vi "MBDRV_Operation.vi"(7 "Unit Address (1)":u8=1, 8 "error in (no error)":errorcluster, 10 "Command List":T4, 11 "VISA resource name":refnum<visa-resource-name>) -> (0 "error out":errorcluster, 2 "Response List":T1, 3 "VISA resource name out":refnum<visa-resource-name>)   [LabVIEW 2010]
uses:
  MBDRV_Command List.ctl
  MBDRV_Command Data.ctl
  MBDRV_Action.ctl
  MBDRV_Response List.ctl
  MBDRV_Response.ctl
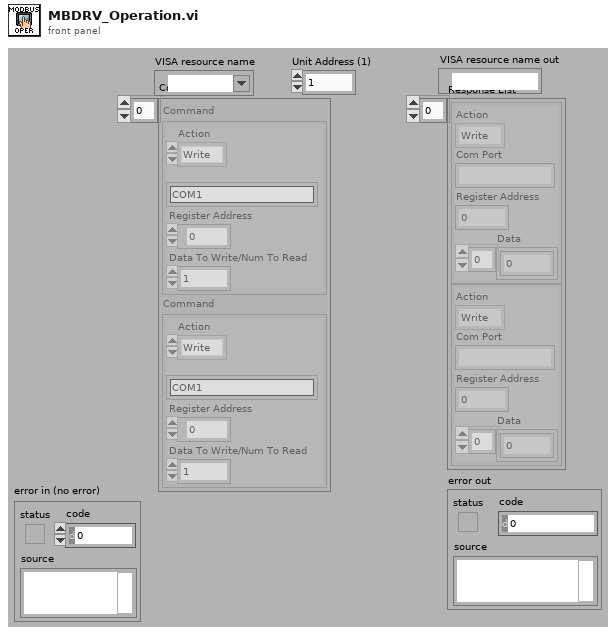
[diagram p1: front panel]
types:
  T1 = typedef "MBDRV_Response List.ctl" = T2[]
  T2 = typedef "MBDRV_Response.ctl" = cluster{"Action":T3, "Com Port":string, "Register Address":u16, "Data":i16[]}
  T3 = typedef "MBDRV_Action.ctl" = enum16{"Write", "Read"}
  T4 = typedef "MBDRV_Command List.ctl" = T5[]
  T5 = typedef "MBDRV_Command Data.ctl" = cluster{"Action":T3, "Com Port":string, "Register Address":u16, "Data To Write/Num To Read":i16}
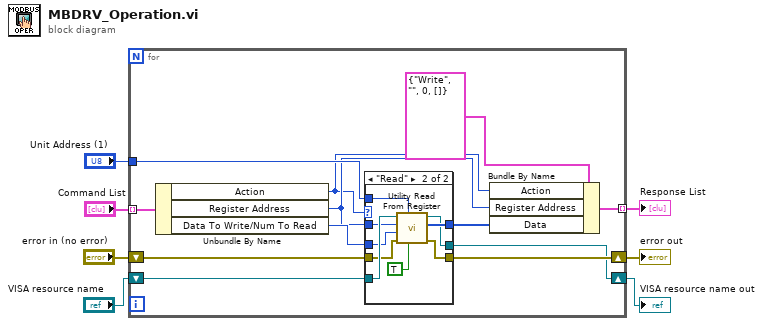
[diagram p0: block diagram]
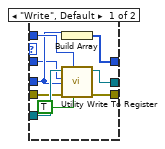
[diagram p2: hidden frame]
diagram:
  n1 = for {
    tunnel: "Unit Address (1)" -> [w14]
    tunnel: "Command List" -> [w19] mode=indexing
    shift-right: [w16] -> w4
    shift-left: "error in (no error)" -> [w17]
    tunnel: [w13] -> w1 mode=indexing
    shift-right: [w11] -> w2
    shift-left: "VISA resource name" -> [w15]
    n2 = Unbundle By Name(w19) -> ("Action"=w8:T3, "Register Address"=w9:u16, "Data To Write/Num To Read"=w18:i16)
    n3 = case shown="\"Read\"" w8 {
      tunnel: w14 -> [w28 w36]
      tunnel: w15 -> [w27 w37]
      tunnel: w9 -> [w21 w30]
      tunnel: w18 -> [w23 w35]
      tunnel: w17 -> [w26 w34]
      tunnel: [w25 w33] -> w16
      tunnel: [w22 w32] -> w10
      tunnel: [w24 w31] -> w11
      frame "Write", Default {
        n4 = Build Array(w23) -> (w22:i16[])
        n5 = call "Utility Write To Register.vi"("Direct Action?"=TRUE, "Unit Address (1)"=w28, "error in (no error)"=w26, "Data (0)"=w23, "Register Address (0)"=w21, "VISA resource name"=w27) -> ("error out"=w25:errorcluster, "VISA resource name out"=w24:refnum<visa-resource-name>)  [unwired: 4 in]
      }
      frame "Read" {
        n6 = call "Utility Read From Register.vi"("Direct Action?"=TRUE, "Unit Address (1)"=w36, "error in (no error)"=w34, "Num Of Reg (1)"=w35, "Register Address (0)"=w30, "VISA resource name"=w37) -> ("error out"=w33:errorcluster, "Data"=w32:i16[], "VISA resource name out"=w31:refnum<visa-resource-name>)  [unwired: 3 in]
      }
    }
    n7 = Bundle By Name(cluster=T2 {"Action"=enum."Write", "Com Port"="", "Register Address"=0, "Data"=[]} ("Response"), "Action"=w8, "Register Address"=w9, "Data"=w10) -> (w13:T2)
  }
  "error out" <- w4
  "Response List" <- w1
  "VISA resource name out" <- w2
